vi "Generate RPC Methods.vi"(7 "RPC Method Parameters":T1[](array[typedef]), 8 "error in (no error)":errorcluster, 11 "Server class in":refnum<vi>) -> (0 "error out":errorcluster, 3 "Server class out":refnum<vi>)   [LabVIEW 2019, in "gRPC Scripting Tools.lvlib"]
uses:
  gRPC Scripting Tools.lvlib
  TypeDefs/RPC Method Parameters.ctl
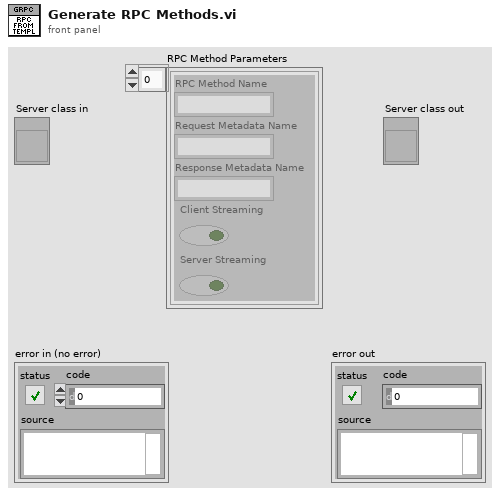
[diagram p1: front panel]
types:
  T1 = typedef "gRPC Scripting Tools.lvlib/RPC Method Parameters.ctl" = cluster{"RPC Method Name":string, "Request Metadata Name":string, "Response Metadata Name":string, "Client Streaming":bool, "Server Streaming":bool}
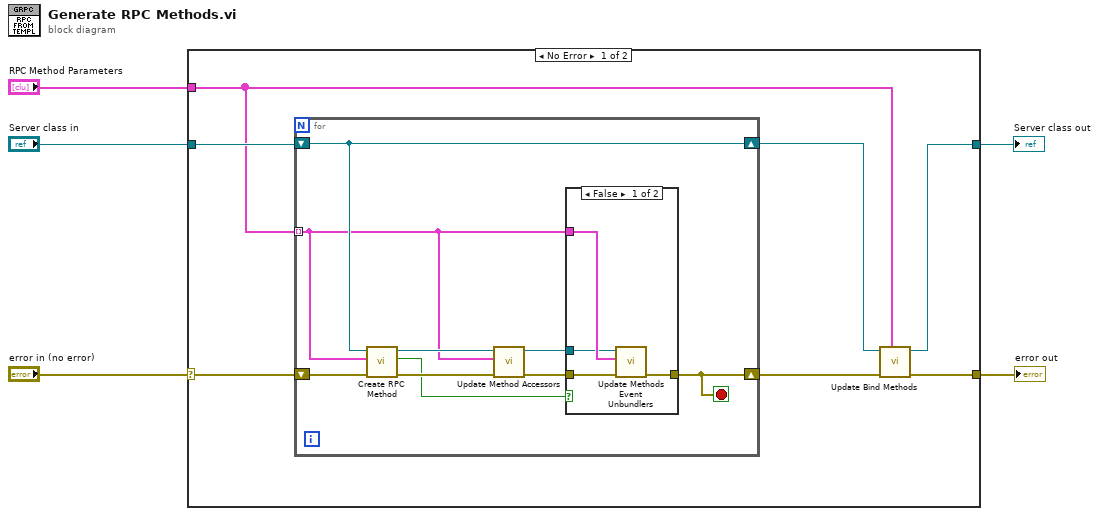
[diagram p0: block diagram]
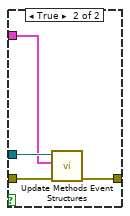
[diagram p2: hidden frame]
diagram:
  n1 = case shown="No Error" "error in (no error)" {
    selector: "error in (no error)" -> [w12 w31]
    tunnel: [w8 w31] -> w5
    tunnel: "Server class in" -> [w11 w30]
    tunnel: [w6 w30] -> w2
    tunnel: "RPC Method Parameters" -> [w9 _]
    frame No Error {
      n2 = for {
        tunnel: w9 -> [w14] mode=indexing
        shift-right: [w20] -> w10
        shift-left: w12 -> [w21]
        shift-right: [w19] -> w7
        shift-left: w11 -> [w19]
        stop <- w20 stop-if-true
        n3 = call "Create RPC Method.vi"("error in (no error)"=w21, "RPC Method Parameters"=w14, "Server class in"=w19) -> ("error out"=w16:errorcluster, "Newly created ?"=w13:bool, "Server class out"=w18:refnum<vi>)  [unwired: 6 in]
        n4 = call "Update Method Accessors.vi"("error in (no error)"=w16, "RPC Method Parameters"=w14, "Server class in"=w18) -> ("error out"=w15:errorcluster, "Server class out"=w17:refnum<vi>)  [unwired: 7 in]
        n5 = case shown="False" w13 {
          tunnel: w15 -> [w25 w29]
          tunnel: w17 -> [w22 w28]
          tunnel: w14 -> [w23 w27]
          tunnel: [w24 w26] -> w20
          frame False {
            n6 = call "Update Methods Event Unbundlers.vi"("error in (no error)"=w25, "RPC Method Parameters"=w23, "LVClassLibrary in"=w22) -> ("error out"=w24:errorcluster)  [unwired: 7 in, 1 out]
          }
          frame True {
            n7 = call "Update Methods Event Structures.vi"("error in (no error)"=w29, "RPC Method Parameters"=w27, "LVClassLibrary in"=w28) -> ("error out"=w26:errorcluster)  [unwired: 7 in, 1 out]
          }
        }
      }
      n8 = call "Update Bind Methods.vi"("RPC Method Parameters"=w9, "error in (no error)"=w10, "Server class in"=w7) -> ("error out"=w8:errorcluster, "Server class out"=w6:refnum<vi>)  [unwired: 7 in]
    }
    frame Error {
    }
  }
  "error out" <- w5
  "Server class out" <- w2
